vi "#FIXME_PFD_Top.vi"(8 "Refresh Rate (Hz)":u32=10, 9 "color_palette":T2={"color1"=16777225, "color2"=16777224, "color_line"=16777225}, 11 "PFD_TopControl":T3={"mav_mode"=1, "ALT"=0.0, "GND ALT"=0.0, "Mission Mode"=21, "Batt Stats"={"Active"=TRUE, "State"=FALSE}, "Sat Stats"={"Active"=TRUE, "State"=FALSE}, "Radio Stats"={"Active"=TRUE, "State"=FALSE}, "Sensor Stats"={"Active"=TRUE, "State"=FALSE}, "SPEED"=0.0, "ASPEED"=0.0, "arm_s"=FALSE}) -> (3 "PFD_Top":picture)   [LabVIEW 2023]
uses:
  <vilib>/Utility/miscctls.llb/LVBoundsTypeDef.ctl
  PFD_Global.vi
panel:
  in  "type":T1(ring)
  in  "stop":bool
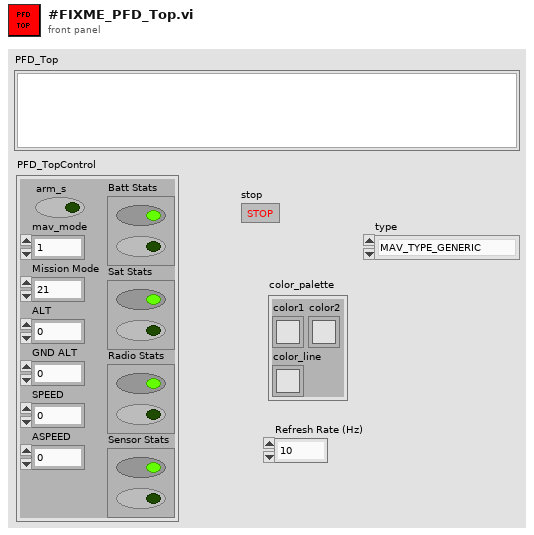
[diagram p1: front panel]
types:
  T1 = enum8{"MAV_TYPE_GENERIC", "MAV_TYPE_FIXED_WING", "MAV_TYPE_QUADROTOR", "MAV_TYPE_COAXIAL", "MAV_TYPE_HELICOPTER", "MAV_TYPE_ANTENNA_TRACKER", "MAV_TYPE_GCS", "MAV_TYPE_AIRSHIP", "MAV_TYPE_FREE_BALLOON", "MAV_TYPE_ROCKET", "MAV_TYPE_GROUND_ROVER", "MAV_TYPE_SURFACE_BOAT", "MAV_TYPE_SUBMARINE", "MAV_TYPE_HEXAROTOR", "MAV_TYPE_OCTOROTOR", "MAV_TYPE_TRICOPTER", "MAV_TYPE_FLAPPING_WING", "MAV_TYPE_KITE", "MAV_TYPE_ONBOARD_CONTROLLER", "MAV_TYPE_VTOL_TAILSITTER_DUOROTOR", "MAV_TYPE_VTOL_TAILSITTER_QUADROTOR", "MAV_TYPE_VTOL_TILTROTOR", "MAV_TYPE_VTOL_FIXEDROTOR", "MAV_TYPE_VTOL_TAILSITTER", "MAV_TYPE_VTOL_TILTWING", "MAV_TYPE_VTOL_RESERVED5", "MAV_TYPE_GIMBAL", "MAV_TYPE_ADSB", "MAV_TYPE_PARAFOIL", "MAV_TYPE_DODECAROTOR", "MAV_TYPE_CAMERA", "MAV_TYPE_CHARGING_STATION", "MAV_TYPE_FLARM", "MAV_TYPE_SERVO", "MAV_TYPE_ODID", "MAV_TYPE_DECAROTOR", "MAV_TYPE_BATTERY", "MAV_TYPE_PARACHUTE", "MAV_TYPE_LOG", "MAV_TYPE_OSD", "MAV_TYPE_IMU", "MAV_TYPE_GPS", "MAV_TYPE_WINCH", "MAV_TYPE_GENERIC_MULTIROTOR", "MAV_TYPE_ILLUMINATOR"}
  T2 = cluster{"color1":u32, "color2":u32, "color_line":u32}
  T3 = cluster{"mav_mode":i16, "ALT":dbl, "GND ALT":dbl, "Mission Mode":i16, "Batt Stats":cluster{"Active":bool, "State":bool}, "Sat Stats":cluster{"Active":bool, "State":bool}, "Radio Stats":cluster{"Active":bool, "State":bool}, "Sensor Stats":cluster{"Active":bool, "State":bool}, "SPEED":dbl, "ASPEED":dbl, "arm_s":bool}
  T4 = typedef "LVBoundsTypeDef.ctl" = cluster{"Width":u32, "Height":u32}
  T5 = cluster{"Font Name:":string, "Size":i16, "Strikeout?":bool, "Italic?":bool, "Underline?":bool, "Outline?":bool, "Shadow?":bool, "Bold?":bool}
  T6 = cluster{"horizontal":enum16{"left", "center", "right"}, "vertical":enum16{"top", "center", "bottom"}}
  T7 = cluster{"left":i16, "top":i16, "right":i16, "bottom":i16}
  T8 = enum16{"User-specified Font", "Application Font", "System Font", "Dialog Font"}
  T9 = typedef "imagedata.ctl" = cluster{"image type":i32, "image depth":i32, "image":u8[], "mask":u8[], "colors":u32[], "Rectangle":cluster{"left":i16, "top":i16, "right":i16, "bottom":i16}}
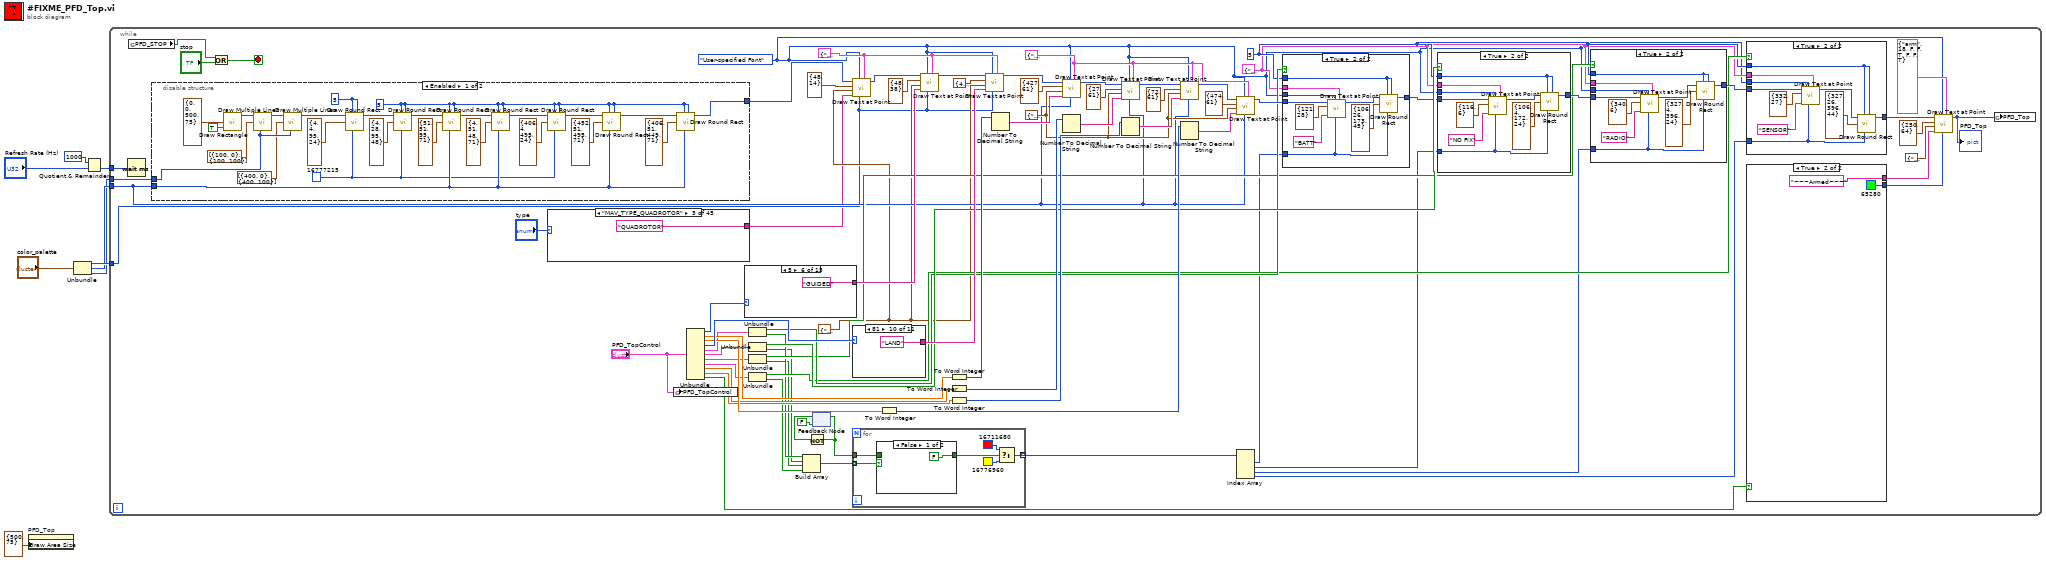
[diagram p0: block diagram]
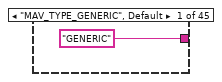
[diagram p2: hidden frame]
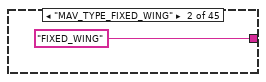
[diagram p3: hidden frame]
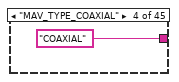
[diagram p4: hidden frame]
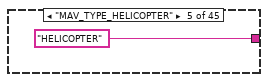
[diagram p5: hidden frame]
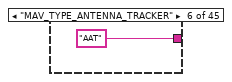
[diagram p6: hidden frame]
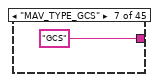
[diagram p7: hidden frame]
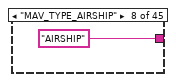
[diagram p8: hidden frame]
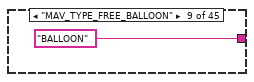
[diagram p9: hidden frame]
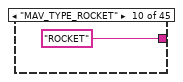
[diagram p10: hidden frame]
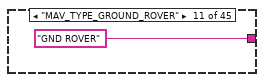
[diagram p11: hidden frame]
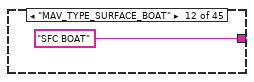
[diagram p12: hidden frame]
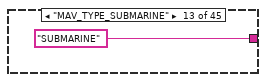
[diagram p13: hidden frame]
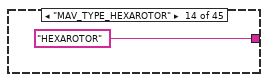
[diagram p14: hidden frame]
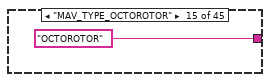
[diagram p15: hidden frame]
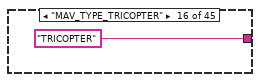
[diagram p16: hidden frame]
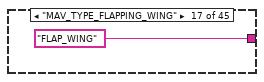
[diagram p17: hidden frame]
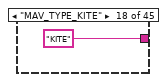
[diagram p18: hidden frame]
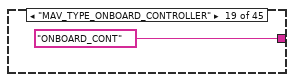
[diagram p19: hidden frame]
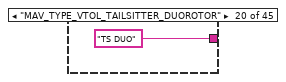
[diagram p20: hidden frame]
diagram:
  n1 = property on="PFD_Top" class="Pict"("Draw Area Size"=T4 {"Width"=500, "Height"=75}) -> ()  [unwired: 2 in, 2 out]
  n2 = Unbundle("color_palette") -> ("color1"=w7:u32, "color2"=w5:u32, "color_line"=w1:u32)
  n3 = Quotient & Remainder(x=u32 1000, y="Refresh Rate (Hz)") -> (floor(x/y)=w2:u32)  [unwired: 1 out]
  n4 = while {
    tunnel: w7 -> [w12]
    tunnel: w5 -> [w18]
    tunnel: w2 -> [w20]
    tunnel: w1 -> [w19]
    stop <- w73 stop-if-true
    w26 = T5 {"Font Name:"="rectangle", "Size"=17, "Strikeout?"=FALSE, "Italic?"=FALSE, "Underline?"=FALSE, "Outline?"=FALSE, "Shadow?"=FALSE, "Bold?"=TRUE} ("[user-specified font] 2")
    w27 = i16 5 ("oval height")
    w15 = T5 {"Font Name:"="rectangle", "Size"=17, "Strikeout?"=FALSE, "Italic?"=FALSE, "Underline?"=FALSE, "Outline?"=FALSE, "Shadow?"=FALSE, "Bold?"=TRUE} ("[user-specified font]")
    w13 = T6 {"horizontal"=enum."center", "vertical"=enum."center"} ("alignment(left, top)")
    w58 = T5 {"Font Name:"="text", "Size"=17, "Strikeout?"=FALSE, "Italic?"=FALSE, "Underline?"=FALSE, "Outline?"=FALSE, "Shadow?"=FALSE, "Bold?"=TRUE} ("[user-specified font]")
    w55 = T6 {"horizontal"=enum."center", "vertical"=enum."center"} ("alignment(left, top)")
    w14 = T8."User-specified Font" ("desired font(Application)")
    n5 = Wait (ms)(milliseconds to wait=w20) -> ()  [unwired: 1 out]
    n6 = global read "PFD_Global.vi" "PFD_STOP"() -> (w74:bool)
    n7 = disable-structure shown="Enabled" {
      disable-tunnel: [w159 w160] -> w17
      disable-tunnel: w19 -> [w158 _]
      disable-tunnel: w18 -> [w157 _]
      frame Enabled {
        w138 = i16 5 ("oval height")
        w134 = u32 16777215 ("color(black)")
        w146 = i16 5 ("oval height")
        n8 = call <vilib>:"Draw Rectangle.vi"("rect"=T7 {"left"=0, "top"=0, "right"=500, "bottom"=75}, "fill?(F)"=TRUE) -> ("new picture"=w142:picture)  [unwired: 7 in]
        n9 = call <vilib>:"Draw Multiple Lines.vi"("picture"=w142, "line endpoints"=cluster{"x":i16, "y":i16}[] [{"x"=100, "y"=0}, {"x"=100, "y"=100}], "color(black)"=w158) -> ("new picture"=w141:picture)  [unwired: 6 in]
        n10 = call <vilib>:"Draw Multiple Lines.vi"("picture"=w141, "line endpoints"=cluster{"x":i16, "y":i16}[] [{"x"=400, "y"=0}, {"x"=400, "y"=100}], "color(black)"=w158) -> ("new picture"=w135:picture)  [unwired: 6 in]
        n11 = call <vilib>:"Draw Round Rect.vi"("picture"=w135, "oval width"=w138, "rect"=T7 {"left"=4, "top"=4, "right"=95, "bottom"=24} ("rect 2"), "color(black)"=w134, "oval height"=w138) -> ("new picture"=w136:picture)  [unwired: 4 in]
        n12 = call <vilib>:"Draw Round Rect.vi"("picture"=w136, "oval width"=w146, "rect"=T7 {"left"=4, "top"=28, "right"=95, "bottom"=48} ("rect 3"), "color(black)"=w134, "oval height"=w146) -> ("new picture"=w155:picture)  [unwired: 4 in]
        n13 = call <vilib>:"Draw Round Rect.vi"("picture"=w155, "oval width"=w146, "rect"=T7 {"left"=51, "top"=51, "right"=95, "bottom"=71} ("rect 4"), "color(black)"=w157, "oval height"=w146) -> ("new picture"=w153:picture)  [unwired: 4 in]
        n14 = call <vilib>:"Draw Round Rect.vi"("picture"=w153, "oval width"=w146, "rect"=T7 {"left"=4, "top"=51, "right"=48, "bottom"=71} ("rect 2"), "color(black)"=w157, "oval height"=w146) -> ("new picture"=w151:picture)  [unwired: 4 in]
        n15 = call <vilib>:"Draw Round Rect.vi"("picture"=w151, "oval width"=w146, "rect"=T7 {"left"=406, "top"=4, "right"=495, "bottom"=24}, "color(black)"=w134, "oval height"=w146) -> ("new picture"=w149:picture)  [unwired: 4 in]
        n16 = call <vilib>:"Draw Round Rect.vi"("picture"=w149, "oval width"=w146, "rect"=T7 {"left"=452, "top"=51, "right"=495, "bottom"=71}, "color(black)"=w157, "oval height"=w146) -> ("new picture"=w147:picture)  [unwired: 4 in]
        n17 = call <vilib>:"Draw Round Rect.vi"("picture"=w147, "oval width"=w146, "rect"=T7 {"left"=406, "top"=51, "right"=449, "bottom"=71} ("rect 3"), "color(black)"=w157, "oval height"=w146) -> ("new picture"=w159:picture)  [unwired: 4 in]
      }
      frame Disabled {
        n18 = call <vilib>:"Flatten Pixmap.vi"("24-bit pixmap"=u32[][] array76x502[38152 elements]) -> ("image data"=w162:T9)  [unwired: 10 in]
        n19 = call <vilib>:"Draw Flattened Pixmap.vi"("image data"=w162) -> ("new picture"=w160:picture)  [unwired: 8 in]
      }
    }
    n20 = Or(x=w74, y="stop") -> (x .or. y?=w73:bool)
    n21 = case shown="\"MAV_TYPE_QUADROTOR\"" "type" {
      tunnel: ["GENERIC" ("text") "FIXED_WING" ("text") "QUADROTOR" ("text") "COAXIAL" ("text") "HELICOPTER" ("text") "AAT" ("text") "GCS" ("text") "AIRSHIP" ("text") "BALLOON" ("text") "ROCKET" ("text") "GND ROVER" ("text") "SFC BOAT" ("text") "SUBMARINE" ("text") "HEXAROTOR" ("text") "OCTOROTOR" ("text") "TRICOPTER" ("text") "FLAP_WING" ("text") "KITE" ("text") "ONBOARD_CONT" ("text") "TS DUO" ("text") "TS QUAD" ("text") "VTOL_TILTROTOR" ("text") "FIXEDROTOR" ("text") "TS VTOL" ("text") "TILTWING" ("text") "" ("text") "GIMBAL" ("text") "ADSB" ("text") "PARAFOIL" ("text") "DODECAROTOR" ("text") "CAMERA" ("text") "STATION" ("text") "FLARM" ("text") "SERVO" ("text") "ODID" ("text") "DECOROTOR" ("text") "BATTERY" ("text") "PARACHUTE" ("text") "LOG" ("text") "OSD" ("text") "IMU" ("text") "GPS" ("text") "WINCH" ("text") "GENERIC M_ROTOR" ("text") "ILLUMINATOR" ("text")] -> w9
      frame "MAV_TYPE_GENERIC", Default {
      }
      frame "MAV_TYPE_FIXED_WING" {
      }
      frame "MAV_TYPE_QUADROTOR" {
      }
      frame "MAV_TYPE_COAXIAL" {
      }
      frame "MAV_TYPE_HELICOPTER" {
      }
      frame "MAV_TYPE_ANTENNA_TRACKER" {
      }
      frame "MAV_TYPE_GCS" {
      }
      frame "MAV_TYPE_AIRSHIP" {
      }
      frame "MAV_TYPE_FREE_BALLOON" {
      }
      frame "MAV_TYPE_ROCKET" {
      }
      frame "MAV_TYPE_GROUND_ROVER" {
      }
      frame "MAV_TYPE_SURFACE_BOAT" {
      }
      frame "MAV_TYPE_SUBMARINE" {
      }
      frame "MAV_TYPE_HEXAROTOR" {
      }
      frame "MAV_TYPE_OCTOROTOR" {
      }
      frame "MAV_TYPE_TRICOPTER" {
      }
      frame "MAV_TYPE_FLAPPING_WING" {
      }
      frame "MAV_TYPE_KITE" {
      }
      frame "MAV_TYPE_ONBOARD_CONTROLLER" {
      }
      frame "MAV_TYPE_VTOL_TAILSITTER_DUOROTOR" {
      }
      frame "MAV_TYPE_VTOL_TAILSITTER_QUADROTOR" {
      }
      frame "MAV_TYPE_VTOL_TILTROTOR" {
      }
      frame "MAV_TYPE_VTOL_FIXEDROTOR" {
      }
      frame "MAV_TYPE_VTOL_TAILSITTER" {
      }
      frame "MAV_TYPE_VTOL_TILTWING" {
      }
      frame "MAV_TYPE_VTOL_RESERVED5" {
      }
      frame "MAV_TYPE_GIMBAL" {
      }
      frame "MAV_TYPE_ADSB" {
      }
      frame "MAV_TYPE_PARAFOIL" {
      }
      frame "MAV_TYPE_DODECAROTOR" {
      }
      frame "MAV_TYPE_CAMERA" {
      }
      frame "MAV_TYPE_CHARGING_STATION" {
      }
      frame "MAV_TYPE_FLARM" {
      }
      frame "MAV_TYPE_SERVO" {
      }
      frame "MAV_TYPE_ODID" {
      }
      frame "MAV_TYPE_DECAROTOR" {
      }
      frame "MAV_TYPE_BATTERY" {
      }
      frame "MAV_TYPE_PARACHUTE" {
      }
      frame "MAV_TYPE_LOG" {
      }
      frame "MAV_TYPE_OSD" {
      }
      frame "MAV_TYPE_IMU" {
      }
      frame "MAV_TYPE_GPS" {
      }
      frame "MAV_TYPE_WINCH" {
      }
      frame "MAV_TYPE_GENERIC_MULTIROTOR" {
      }
      frame "MAV_TYPE_ILLUMINATOR" {
      }
    }
    n22 = global write "PFD_Global.vi" "PFD_TopControl"("PFD_TopControl") -> ()
    n23 = Unbundle("PFD_TopControl") -> ("mav_mode"=w88:i16, "ALT"=w86:dbl, "GND ALT"=w85:dbl, "Mission Mode"=w87:i16, "Batt Stats"=w79:cluster{"Active":bool, "State":bool}, "Sat Stats"=w80:cluster{"Active":bool, "State":bool}, "Radio Stats"=w81:cluster{"Active":bool, "State":bool}, "Sensor Stats"=w82:cluster{"Active":bool, "State":bool}, "SPEED"=w84:dbl, "ASPEED"=w83:dbl, "arm_s"=w76:bool)
    n24 = case shown="5" w88 {
      tunnel: ["" "STAB" ("text") "ACRO" ("text") "HOLD" ("text") "AUTO" ("text") "GUIDED" ("text") "LOITER" ("text") "RTL" ("text") "CIRCLE" ("text") "LAND" ("text") "OF LOI" ("text") "DRIFT" ("text") "SPORT" ("text") "HYBRID" ("text") "TAOFF" ("text")] -> w52
      frame 0, Default {
      }
      frame 1 {
      }
      frame 2 {
      }
      frame 3 {
      }
      frame 4 {
      }
      frame 5 {
      }
      frame 6 {
      }
      frame 7 {
      }
      frame 8 {
      }
      frame 9 {
      }
      frame 10 {
      }
      frame 11 {
      }
      frame 12 {
      }
      frame 13 {
      }
      frame 22 {
      }
    }
    n25 = Unbundle(w79) -> ("Active"=w46:bool, "State"=w40:bool)
    n26 = Unbundle(w80) -> ("Active"=w47:bool, "State"=w39:bool)
    n27 = Unbundle(w81) -> ("Active"=w43:bool, "State"=w38:bool)
    n28 = Unbundle(w82) -> ("Active"=w41:bool, "State"=w37:bool)
    n29 = Build Array(w40, w39, w38, w37) -> (w36:bool[])
    n30 = feedback #1(FALSE) -> (w31:bool)
    n31 = Not(x=w31) -> (.not. x?=w30:bool)
    n32 = feedback-in #1(w30) -> ()
    n33 = call <vilib>:"Draw Text at Point.vi"("[user-specified font]"=w15, "text color(black)"=w12, "desired font(Application)"=w14, "text"=w9, "alignment(left, top)"=w13, "origin"=cluster{"x":i16, "y":i16} {"x"=48, "y"=14}, "picture"=w17) -> ("new picture"=w16:picture)  [unwired: 3 in, 1 out]
    n34 = case shown="81" w87 {
      tunnel: ["" "NAV" ("text") "LOITER" ("text") "LOITER" ("text") "LOITER" ("text") " RTL" ("text") "LAND" ("text") "TAOFF" ("text") " ROI" ("text") "LAND" ("text") "NAV" ("text")] -> w50
      frame 0, Default {
      }
      frame 16 {
      }
      frame 17 {
      }
      frame 18 {
      }
      frame 19 {
      }
      frame 20 {
      }
      frame 21 {
      }
      frame 22 {
      }
      frame 80 {
      }
      frame 81 {
      }
      frame 82 {
      }
    }
    n35 = for {
      tunnel: w36 -> [w169] mode=indexing
      tunnel: [w168] -> w29 mode=indexing
      tunnel: w30 -> [w167]
      n36 = case shown="False" w169 {
        tunnel: [FALSE w174] -> w170
        tunnel: w167 -> [_ w174]
        frame False {
        }
        frame True {
        }
      }
      n37 = Select(t=u32 16711680 ("color(black)"), s=w170, f=u32 16776960 ("color(black)")) -> (s? t:f=w168:u32)
    }
    n38 = To Word Integer(number=w85) -> (16bit integer=w56:i16)
    n39 = call <vilib>:"Draw Text at Point.vi"("[user-specified font]"=w15, "text color(black)"=w12, "desired font(Application)"=w14, "text"=w52, "alignment(left, top)"=w13, "origin"=cluster{"x":i16, "y":i16} {"x"=48, "y"=38} ("origin 3"), "picture"=w16) -> ("new picture"=w51:picture)  [unwired: 3 in, 1 out]
    n40 = To Word Integer(number=w86) -> (16bit integer=w66:i16)
    n41 = To Word Integer(number=w84) -> (16bit integer=w65:i16)
    n42 = To Word Integer(number=w83) -> (16bit integer=w62:i16)
    n43 = call <vilib>:"Draw Text at Point.vi"("[user-specified font]"=w15, "text color(black)"=w12, "desired font(Application)"=w14, "text"=w50, "alignment(left, top)"=w13, "origin"=cluster{"x":i16, "y":i16} {"x"=448, "y"=14} ("origin 2"), "picture"=w51) -> ("new picture"=w48:picture)  [unwired: 3 in, 1 out]
    n44 = Number To Decimal String(number=w66) -> (decimal integer string=w70:string)  [unwired: 1 in]
    n45 = call <vilib>:"Draw Text at Point.vi"("[user-specified font]"=w58, "text color(black)"=w18, "desired font(Application)"=w14, "text"=w70, "alignment(left, top)"=w55, "origin"=cluster{"x":i16, "y":i16} {"x"=427, "y"=61}, "picture"=w48) -> ("new picture"=w61:picture)  [unwired: 3 in, 1 out]
    n46 = Number To Decimal String(number=w65) -> (decimal integer string=w68:string)  [unwired: 1 in]
    n47 = call <vilib>:"Draw Text at Point.vi"("[user-specified font]"=w58, "text color(black)"=w18, "desired font(Application)"=w14, "text"=w68, "alignment(left, top)"=w55, "origin"=cluster{"x":i16, "y":i16} {"x"=27, "y"=61} ("origin 2"), "picture"=w61) -> ("new picture"=w60:picture)  [unwired: 3 in, 1 out]
    n48 = Number To Decimal String(number=w62) -> (decimal integer string=w63:string)  [unwired: 1 in]
    n49 = call <vilib>:"Draw Text at Point.vi"("[user-specified font]"=w58, "text color(black)"=w18, "desired font(Application)"=w14, "text"=w63, "alignment(left, top)"=w55, "origin"=cluster{"x":i16, "y":i16} {"x"=72, "y"=61} ("origin 3"), "picture"=w60) -> ("new picture"=w59:picture)  [unwired: 3 in, 1 out]
    n50 = Number To Decimal String(number=w56) -> (decimal integer string=w57:string)  [unwired: 1 in]
    n51 = call <vilib>:"Draw Text at Point.vi"("[user-specified font]"=w58, "text color(black)"=w18, "desired font(Application)"=w14, "text"=w57, "alignment(left, top)"=w55, "origin"=cluster{"x":i16, "y":i16} {"x"=474, "y"=61}, "picture"=w59) -> ("new picture"=w78:picture)  [unwired: 3 in, 1 out]
    n52 = Index Array(array=w29) -> (element #1=w35:u32, element #2=w34:u32, element #3=w33:u32, element #4=w32:u32)  [unwired: 4 in]
    n53 = case shown="True" w46 {
      tunnel: w78 -> [w197 w199]
      tunnel: w14 -> [_ w205]
      tunnel: [w197 w206] -> w45
      tunnel: w27 -> [_ w201]
      tunnel: w26 -> [_ w200]
      tunnel: w35 -> [_ w198]
      frame False {
      }
      frame True {
        n54 = call <vilib>:"Draw Text at Point.vi"("[user-specified font]"=w200, "text color(black)"=w198, "desired font(Application)"=w205, "text"="BATT", "origin"=cluster{"x":i16, "y":i16} {"x"=121, "y"=28} ("origin 2"), "picture"=w199) -> ("new picture"=w207:picture)  [unwired: 4 in, 1 out]
        n55 = call <vilib>:"Draw Round Rect.vi"("picture"=w207, "oval width"=w201, "rect"=T7 {"left"=106, "top"=26, "right"=173, "bottom"=45}, "color(black)"=w198, "oval height"=w201) -> ("new picture"=w206:picture)  [unwired: 4 in]
      }
    }
    n56 = case shown="True" w47 {
      tunnel: [w208 w217] -> w44
      tunnel: w14 -> [_ w216]
      tunnel: w26 -> [_ w212]
      tunnel: w45 -> [w208 w211]
      tunnel: w27 -> [_ w210]
      tunnel: w34 -> [_ w209]
      frame False {
      }
      frame True {
        n57 = call <vilib>:"Draw Text at Point.vi"("[user-specified font]"=w212, "text color(black)"=w209, "desired font(Application)"=w216, "text"="NO FIX", "origin"=cluster{"x":i16, "y":i16} {"x"=116, "y"=6}, "picture"=w211) -> ("new picture"=w218:picture)  [unwired: 4 in, 1 out]
        n58 = call <vilib>:"Draw Round Rect.vi"("picture"=w218, "oval width"=w210, "rect"=T7 {"left"=106, "top"=4, "right"=172, "bottom"=24} ("rect 2"), "color(black)"=w209, "oval height"=w210) -> ("new picture"=w217:picture)  [unwired: 4 in]
      }
    }
    n59 = case shown="True" w43 {
      tunnel: w44 -> [w186 w189]
      tunnel: [w186 w187] -> w42
      tunnel: w27 -> [_ w196]
      tunnel: w14 -> [_ w195]
      tunnel: w26 -> [_ w191]
      tunnel: w33 -> [_ w190]
      frame False {
      }
      frame True {
        n60 = call <vilib>:"Draw Text at Point.vi"("[user-specified font]"=w191, "text color(black)"=w190, "desired font(Application)"=w195, "text"="RADIO", "origin"=cluster{"x":i16, "y":i16} {"x"=340, "y"=6} ("origin 2"), "picture"=w189) -> ("new picture"=w188:picture)  [unwired: 4 in, 1 out]
        n61 = call <vilib>:"Draw Round Rect.vi"("picture"=w188, "oval width"=w196, "rect"=T7 {"left"=327, "top"=4, "right"=396, "bottom"=24}, "color(black)"=w190, "oval height"=w196) -> ("new picture"=w187:picture)  [unwired: 4 in]
      }
    }
    n62 = case shown="True" w41 {
      tunnel: w42 -> [w175 w178]
      tunnel: [w175 w176] -> w77
      tunnel: w27 -> [_ w185]
      tunnel: w14 -> [_ w179]
      tunnel: w26 -> [_ w181]
      tunnel: w32 -> [_ w180]
      frame False {
      }
      frame True {
        n63 = call <vilib>:"Draw Text at Point.vi"("[user-specified font]"=w181, "text color(black)"=w180, "desired font(Application)"=w179, "text"="SENSOR", "origin"=cluster{"x":i16, "y":i16} {"x"=332, "y"=27} ("origin 3"), "picture"=w178) -> ("new picture"=w177:picture)  [unwired: 4 in, 1 out]
        n64 = call <vilib>:"Draw Round Rect.vi"("picture"=w177, "oval width"=w185, "rect"=T7 {"left"=327, "top"=26, "right"=396, "bottom"=44}, "color(black)"=w180, "oval height"=w185) -> ("new picture"=w176:picture)  [unwired: 4 in]
      }
    }
    n65 = case shown="True" w76 {
      tunnel: ["~~~Disarmed~~~" ("text 2") "~~~Armed~~~" ("text")] -> w23
      tunnel: [u32 16711680 ("text color(black)") u32 65280 ("text color(black)")] -> w22
      frame False {
      }
      frame True {
      }
    }
    n66 = call <vilib>:"Draw Text at Point.vi"("[user-specified font]"=T5 {"Font Name:"="arm", "Size"=18, "Strikeout?"=FALSE, "Italic?"=FALSE, "Underline?"=TRUE, "Outline?"=FALSE, "Shadow?"=FALSE, "Bold?"=TRUE}, "text color(black)"=w22, "desired font(Application)"=w14, "text"=w23, "alignment(left, top)"=T6 {"horizontal"=enum."center", "vertical"=enum."center"}, "origin"=cluster{"x":i16, "y":i16} {"x"=250, "y"=64}, "picture"=w77) -> ("new picture"=w72:picture)  [unwired: 3 in, 1 out]
    "PFD_Top" <- w72
    n67 = global write "PFD_Global.vi" "PFD_Top"(w72) -> ()
  }
